vi "Swerve Wheel.vi"(4 "Inputs":dbl[](array[numeric])=[-0.0, -0.0, 0.0, 0.0, 0.0, 14.0, 19.623009453190406, 13.75], 5 "Wheel":T1(ring)=enum."Front Left") -> (0 "Speed":dbl, 1 "Spin Motor Power":dbl)   [LabVIEW 2016]
doc: "Used within Swerve Drive.vi.\nControls an individual wheel."
uses:
  Drive Globals.vi
panel:
  out "PID Tracking":cluster{"Goal Wheel Position":dbl, dbl}(graph)={"Goal Wheel Position"=0.0, -90.17571233858979}
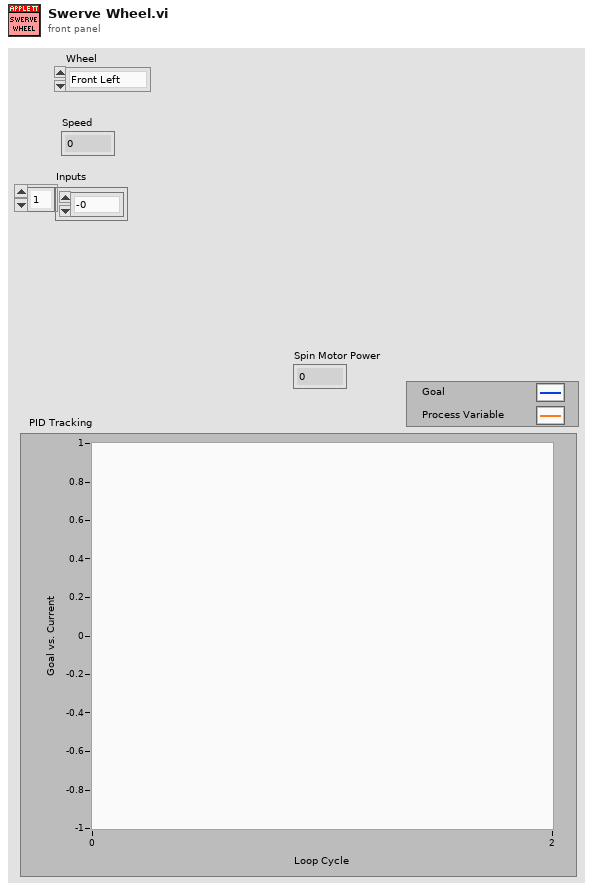
[diagram p1: front panel]
types:
  T1 = enum16{"Back Left", "Back Right", "Front Left", "Front Right"}
  T2 = enum16{"Z", "Y", "X", "Rot. Point X", "Rot. Point Y", "Width/2", "Max", "Length/2"}
  T3 = enum16{"Z Axis", "Y", "X", "Rot. Point X", "Rot. Point Y", "Width/2", "Max", "Length/2"}
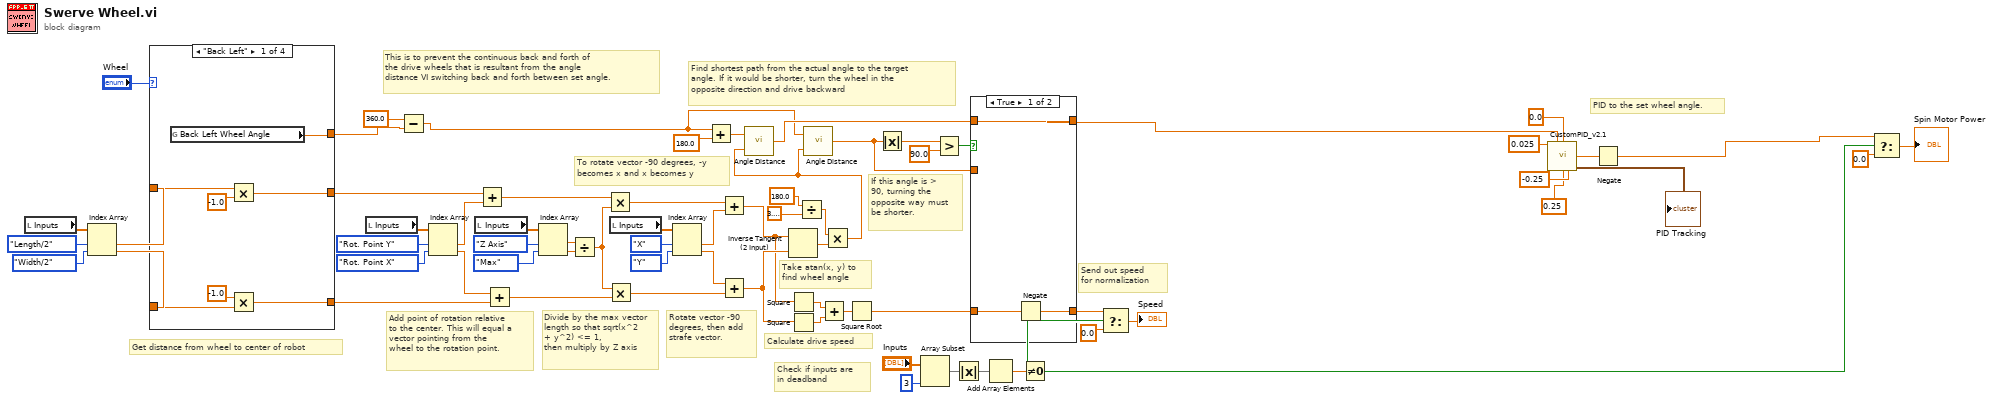
[diagram p0: block diagram]
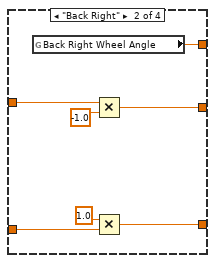
[diagram p3: hidden frame]
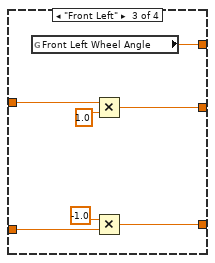
[diagram p4: hidden frame]
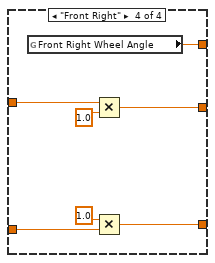
[diagram p5: hidden frame]
diagram:
  # "PID to the set wheel angle."
  # "This is to prevent the continuous back and forth of \nthe drive wheels that is resultant from the angle \ndistance VI switching back and forth between set angle."
  # "To rotate vector -90 degrees, -y becomes x and x becomes y"
  # "Divide by the max vector length so that sqrt(x^2 + y^2) <= 1,\nthen multiply by Z axis"
  # "Add point of rotation relative to the center. This will equal a vector pointing from the\nwheel to the rotation point."
  # "Send out speed\nfor normalization"
  # "Check if inputs are\nin deadband"
  # "If this angle is > 90, turning the opposite way must be shorter."
  # "Find shortest path from the actual angle to the target angle. If it would be shorter, turn the wheel in the opposite direction and drive backward"
  # "Take atan(x, y) to find wheel angle"
  # "Calculate drive speed"
  # "Rotate vector -90 degrees, then add strafe vector."
  # "Get distance from wheel to center of robot"
  n1 = local read "Inputs"() -> (w22:dbl[])
  n2 = Index Array(array=w22, index #1=T2."Length/2", index #2=T2."Width/2") -> (element #1=w21:dbl, element #2=w20:dbl)
  n3 = case shown="\"Back Left\"" "Wheel" {
    tunnel: w21 -> [w74 w81 w88 w95]
    tunnel: w20 -> [w72 w79 w86 w93]
    tunnel: [w71 w78 w85 w92] -> w45
    tunnel: [w70 w77 w84 w91] -> w41
    tunnel: [w69 w76 w83 w90] -> w11
    frame "Back Left" {
      n4 = global read "Drive Globals.vi" "Back Left Wheel Angle"() -> (w69:dbl)
      n5 = Multiply(x=w74, y=-1.0) -> (x*y=w71:dbl)
      n6 = Multiply(x=-1.0 ("y"), y=w72) -> (x*y=w70:dbl)
    }
    frame "Back Right" {
      n7 = global read "Drive Globals.vi" "Back Right Wheel Angle"() -> (w76:dbl)
      n8 = Multiply(x=w81, y=-1.0) -> (x*y=w78:dbl)
      n9 = Multiply(x=1.0 ("y"), y=w79) -> (x*y=w77:dbl)
    }
    frame "Front Left" {
      n10 = global read "Drive Globals.vi" "Front Left Wheel Angle"() -> (w83:dbl)
      n11 = Multiply(x=w88, y=1.0) -> (x*y=w85:dbl)
      n12 = Multiply(x=-1.0 ("y"), y=w86) -> (x*y=w84:dbl)
    }
    frame "Front Right" {
      n13 = global read "Drive Globals.vi" "Front Right Wheel Angle"() -> (w90:dbl)
      n14 = Multiply(x=w95, y=1.0) -> (x*y=w92:dbl)
      n15 = Multiply(x=1.0 ("y"), y=w93) -> (x*y=w91:dbl)
    }
  }
  n16 = local read "Inputs"() -> (w43:dbl[])
  n17 = Subtract(x=360.0, y=w11) -> (x-y=w10:dbl)
  n18 = Index Array(array=w43, index #1=T2."Rot. Point Y", index #2=T2."Rot. Point X") -> (element #1=w39:dbl, element #2=w40:dbl)
  n19 = local read "Inputs"() -> (w37:dbl[])
  n20 = Add(x=w45, y=w39) -> (x+y=w19:dbl)
  n21 = Add(x=w40, y=w41) -> (x+y=w33:dbl)
  n22 = Index Array(array=w37, index #1=T3."Z Axis", index #2=T2."Max") -> (element #1=w34:dbl, element #2=w35:dbl)
  n23 = Divide(x=w34, y=w35) -> (x/y=w32:dbl)
  n24 = Multiply(x=w19, y=w32) -> (x*y=w16:dbl)
  n25 = Multiply(x=w32, y=w33) -> (x*y=w27:dbl)
  n26 = local read "Inputs"() -> (w30:dbl[])
  n27 = Index Array(array=w30, index #1=T2."X", index #2=T2."Y") -> (element #1=w25:dbl, element #2=w26:dbl)
  n28 = Add(x=w10, y=180.0 ("f")) -> (x+y=w53:dbl)
  n29 = Add(x=w16, y=w25) -> (x+y=w23:dbl)
  n30 = Add(x=w26, y=w27) -> (x+y=w24:dbl)
  n31 = Inverse Tangent (2 Input)(1:w24, 2:w23) -> (0:w65:dbl)
  n32 = Square(x=w23) -> (x^2=w28:dbl)
  n33 = Square(x=w24) -> (x^2=w64:dbl)
  n34 = Divide(x=180.0 ("y"), y=3.141592653589793) -> (x/y=w62:dbl)
  n35 = Add(x=w28, y=w64) -> (x+y=w63:dbl)
  n36 = Multiply(x=w62, y=w65) -> (x*y=w15:dbl)
  n37 = call "Angle Distance.vi"("target angle"=w15, "current angle"=w53) -> ("distance"=w17:dbl)
  n38 = call "Angle Distance.vi"("target angle"=w15, "current angle"=w10) -> ("distance"=w56:dbl)
  n39 = Square Root(x=w63) -> (sqrt(x)=w55:dbl)
  n40 = Absolute Value(x=w56) -> (abs(x)=w57:dbl)
  n41 = Array Subset(array="Inputs", length=3) -> (w52:dbl[])  [unwired: 1 in]
  n42 = Greater?(x=w57, y=90.0) -> (0:w48:bool)
  n43 = Absolute Value(x=w52) -> (abs(x)=w46:dbl[])
  n44 = case shown="True" w48 {
    tunnel: w17 -> [w99 _]
    tunnel: w56 -> [_ w101]
    tunnel: [w97 w100] -> w51
    tunnel: w55 -> [w98 w100]
    tunnel: [w99 w101] -> w13
    frame True {
      n45 = Negate(x=w98) -> (-x=w97:dbl)
    }
    frame False {
    }
  }
  n46 = Add Array Elements(numeric array=w46) -> (sum=w66:dbl)
  n47 = Not Equal To 0?(x=w66) -> (x != 0?=w47:bool)
  n48 = Select(t=w51, s=w47, f=0.0) -> (s? t:f=→"Speed":dbl)
  n49 = call "CustomPID_v2.1.vi"("Kp"=0.025, "Process Variable"=w13, "Goal"=0.0, "Max Ouput"=0.25, "Min Output"=-0.25) -> ("Command"=w5:dbl, "PID Tracking"=→"PID Tracking":cluster{"Goal Wheel Position":dbl, dbl})  [unwired: 8 in, 1 out]
  n50 = Negate(x=w5) -> (-x=w12:dbl)
  n51 = Select(t=w12, s=w47, f=0.0) -> (s? t:f=→"Spin Motor Power":dbl)
